vi "Copy of TempControl.vi"() -> ()   [LabVIEW 2015]
uses:
  <vilib>/addons/control/pid/NI_PID_pid.lvlib
  <vilib>/addons/control/pid/pid.llb/PID (DBL).vi
  <vilib>/addons/control/pid/pid.llb/PID Control Input Filter (DBL).vi
  <vilib>/addons/control/pid/pid.llb/PID Output Rate Limiter (DBL).vi
panel:
  out "String":string
  in  "output rate (EGU/min)":dbl=1.0 format="%.2f"
  out "Waveform Chart":cluster{"output":dbl, "Numeric":dbl}(graph)
  in  "Param":sgl[](array[numeric])
  in  "process variable":dbl format="%.2f"
  in  "dt (s)":dbl=-1.0 format="%.3f"
  in  "Bool":bool
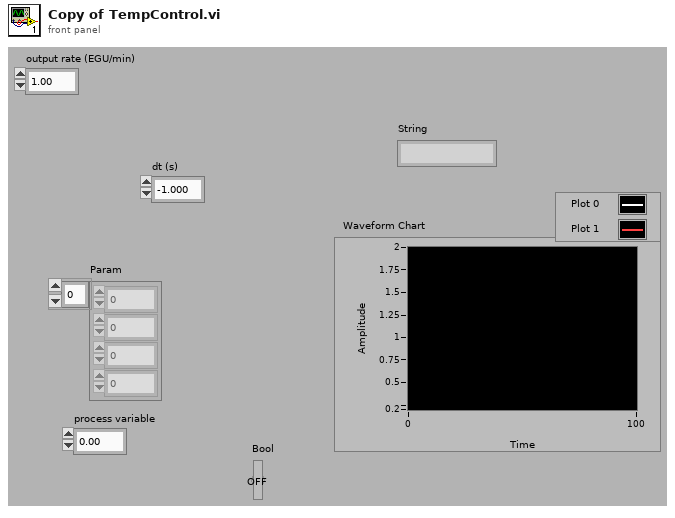
[diagram p1: front panel]
types:
  T1 = cluster{"Numeric":dbl, "Numeric":dbl, "Numeric":dbl}
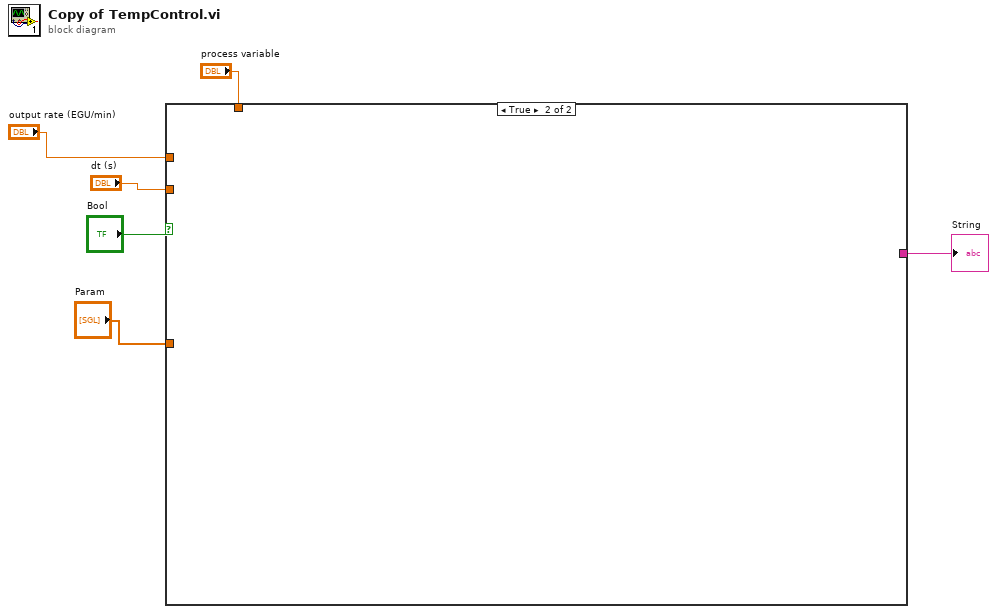
[diagram p0: block diagram]
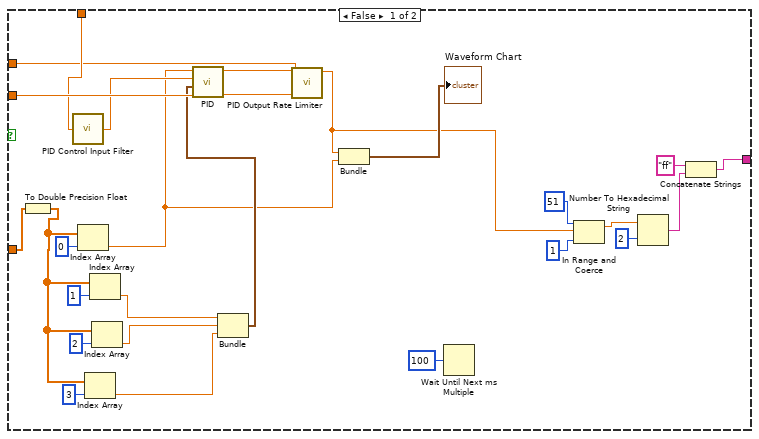
[diagram p2: hidden frame]
diagram:
  n1 = case shown="True" "Bool" {
    tunnel: "dt (s)" -> [w33 _]
    tunnel: "process variable" -> [w32 _]
    tunnel: "Param" -> [w14 _]
    tunnel: "output rate (EGU/min)" -> [w20 _]
    tunnel: [w7 _] -> w1
    frame False {
      n2 = To Double Precision Float(number=w14) -> (double precision float=w13:dbl[])
      n3 = call-poly <vilib>:"PID Control Input Filter.vi"("input"=w32) -> ("output"=w31:dbl)  [unwired: 4 in]
      n4 = Index Array(array=w13, index=0) -> (element=w18:dbl)
      n5 = Index Array(array=w13, index=3) -> (element=w24:dbl)
      n6 = Index Array(array=w13, index=1) -> (element=w26:dbl)
      n7 = Index Array(array=w13, index=2) -> (element=w25:dbl)
      n8 = Bundle("Numeric"=w26, "Numeric"=w25, "Numeric"=w24) -> (w23:T1)  [unwired: 1 in]
      n9 = call-poly <vilib>:"PID.vi"("dt (s)"=w33, "PID gains"=w23, "process variable"=w31, "setpoint"=w18) -> ("dt out (s)"=w21:dbl, "output"=w22:dbl)  [unwired: 6 in]
      n10 = call-poly <vilib>:"PID Output Rate Limiter.vi"("dt (s)"=w21, "output rate (EGU/min)"=w20, "input (controller output)"=w22) -> ("output"=w12:dbl)  [unwired: 5 in, 1 out]
      n11 = Bundle("output"=w12, "Numeric"=w18) -> (→"Waveform Chart":cluster{"output":dbl, "Numeric":dbl})  [unwired: 1 in]
      n12 = Wait Until Next ms Multiple(millisecond multiple=u32 100) -> ()  [unwired: 1 out]
      n13 = In Range and Coerce(upper limit=i8 51, x=w12, lower limit=i8 1) -> (coerced(x)=w11:dbl)  [unwired: 1 out]
      n14 = Number To Hexadecimal String(1:i16 2 ("width (-)"), 2:w11) -> (0:w8:string)
      n15 = Concatenate Strings("ff" ("string"), w8) -> (w7:string)
    }
    frame True {
    }
  }
  "String" <- w1
